vi "ID_Connection.vi"(11 "error in":errorcluster) -> (4 "Arduino":refnum<visa-resource-name>, 6 "Arduino":bool, 8 "Pump":refnum<visa-resource-name>, 10 "Pump":bool)   [LabVIEW 2022 SP3]
uses:
  <vilib>/Instr/_visa.llb/VISA Find Search Mode.ctl
  <vilib>/Instr/_visa.llb/VISA Configure Serial Port (Instr).vi
  <vilib>/regexp/Match Regular Expression.xnode
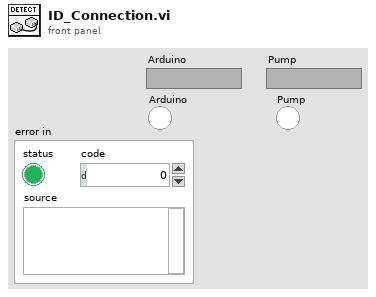
[diagram p1: front panel]
types:
  T1 = typedef "VISA Find Search Mode.ctl" = u32
  T2 = cluster{"VISA resource name":refnum<visa-resource-name>, "error out":errorcluster}
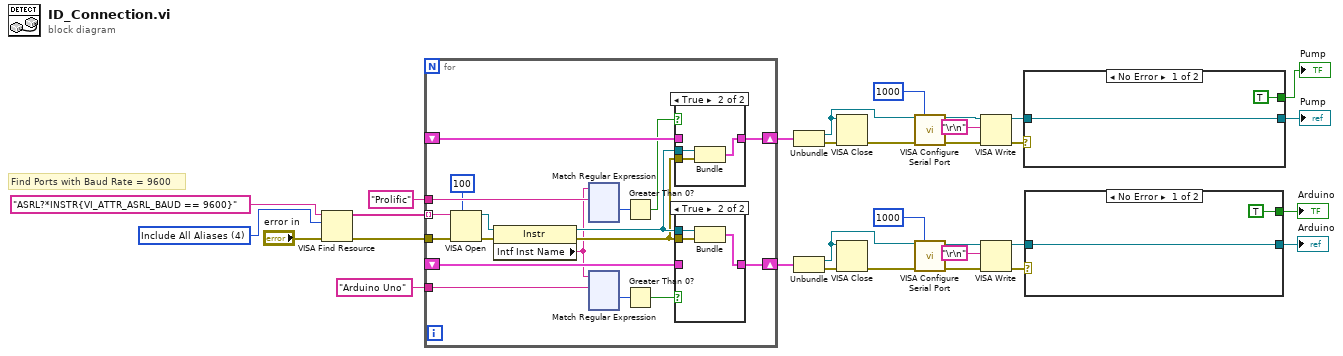
[diagram p0: block diagram]
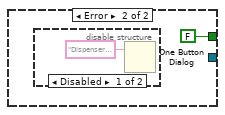
[diagram p2: hidden frame]
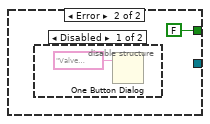
[diagram p4: hidden frame]
diagram:
  w20 = T1 4 items=["Canonical Names Only"=0, "Aliases Only"=2, "Include Matching Aliases"=3, "Include All Aliases"=4] ("Search Mode")
  # "Find Ports with Baud Rate = 9600"
  n1 = VISA Find Resource(8:"error in", 10:w20, 11:"ASRL?*INSTR{VI_ATTR_ASRL_BAUD == 9600}" ("expression (\"?*\")")) -> (0:w28:errorcluster, 3:w31:string[])  [unwired: 1 out]
  n2 = for {
    tunnel: w31 -> [w49] mode=indexing
    tunnel: "Arduino Uno" -> [w45]
    shift-right: [w43] -> w30
    shift-left: _ -> [w42]
    tunnel: w28 -> [w41]
    shift-right: [w40] -> w14
    shift-left: _ -> [w39]
    tunnel: "Prolific" -> [w34]
    n3 = VISA Open(timeout (0)=u32 100 ("VISA Open timeout (0)"), error in (no error)=w41, VISA resource name=w49) -> (VISA resource name=w48:refnum<visa-resource-name>, error out=w44:errorcluster)  [unwired: 2 in]
    n4 = property class="Instr"(reference=w48, error in=w44) -> (reference out=w36:refnum<visa-resource-name>, error out=w35:errorcluster, "Intf Inst Name"=w33:string)
    n5 = xnode "Match Regular Expression"("input string"=w33, "regular expression"=w34) -> ("offset past match"=w38:i32)  [unwired: 4 in, 4 out]
    n6 = xnode "Match Regular Expression"("input string"=w33, "regular expression"=w45) -> ("offset past match"=w47:i32)  [unwired: 4 in, 4 out]
    n7 = Greater Than 0?(x=w38) -> (x > 0?=w37:bool)
    n8 = Greater Than 0?(x=w47) -> (x > 0?=w46:bool)
    n9 = case shown="True" w37 {
      tunnel: w36 -> [_ w170]
      tunnel: w35 -> [_ w169]
      tunnel: [w167 w168] -> w40
      tunnel: w39 -> [w167 _]
      frame False {
      }
      frame True {
        n10 = Bundle("VISA resource name"=w170, "error out"=w169) -> (w168:T2)  [unwired: 1 in]
      }
    }
    n11 = case shown="True" w46 {
      tunnel: w36 -> [_ w174]
      tunnel: w35 -> [_ w173]
      tunnel: [w171 w172] -> w43
      tunnel: w42 -> [w171 _]
      frame False {
      }
      frame True {
        n12 = Bundle("VISA resource name"=w174, "error out"=w173) -> (w172:T2)  [unwired: 1 in]
      }
    }
  }
  n13 = Unbundle(w14) -> ("VISA resource name"=w12:refnum<visa-resource-name>, "error out"=w13:errorcluster)
  n14 = Unbundle(w30) -> ("VISA resource name"=w21:refnum<visa-resource-name>, "error out"=w25:errorcluster)
  n15 = VISA Close(VISA resource name=w12, error in (no error)=w13) -> (error out=w17:errorcluster)
  n16 = VISA Close(VISA resource name=w21, error in (no error)=w25) -> (error out=w24:errorcluster)
  n17 = call-poly "VISA Configure Serial Port"("VISA resource name"=w12, "timeout (10sec)"=u32 1000, "error in (no error)"=w17) -> ("VISA resource name out"=w16:refnum<visa-resource-name>, "error out"=w15:errorcluster)  [unwired: 11 in]
  n18 = call-poly "VISA Configure Serial Port"("VISA resource name"=w21, "timeout (10sec)"=u32 1000, "error in (no error)"=w24) -> ("VISA resource name out"=w23:refnum<visa-resource-name>, "error out"=w22:errorcluster)  [unwired: 11 in]
  n19 = VISA Write(VISA resource name=w16, write buffer="\r\n", error in (no error)=w15) -> (VISA resource name out=w5:refnum<visa-resource-name>, error out=w7:errorcluster)  [unwired: 1 out]
  n20 = VISA Write(VISA resource name=w23, write buffer="\r\n", error in (no error)=w22) -> (VISA resource name out=w11:refnum<visa-resource-name>, error out=w10:errorcluster)  [unwired: 1 out]
  n21 = case shown="No Error" w7 {
    tunnel: [w293 _] -> w6
    tunnel: w5 -> [w293 _]
    tunnel: [TRUE FALSE] -> w4
    frame No Error {
    }
    frame Error {
      n22 = disable-structure shown="Disabled" {
        frame Disabled {
          n23 = One Button Dialog(message="Dispenser Connection Error!") -> ()  [unwired: 1 in, 1 out]
        }
        frame Enabled {
        }
      }
    }
  }
  "Pump" <- w6
  "Pump" <- w4
  n24 = case shown="No Error" w10 {
    tunnel: [TRUE FALSE] -> w8
    tunnel: w11 -> [w296 _]
    tunnel: [w296 _] -> w9
    frame No Error {
    }
    frame Error {
      n25 = disable-structure shown="Disabled" {
        frame Disabled {
          n26 = One Button Dialog(message="Valve Connection Error!") -> ()  [unwired: 1 in, 1 out]
        }
        frame Enabled {
        }
      }
    }
  }
  "Arduino" <- w9
  "Arduino" <- w8
